vi "LabVIEWSensorDisplayandDrillControlRev1.0.0.vi"() -> ()   [LabVIEW 2020]
uses:
  <vilib>/Instr/_visa.llb/VISA Configure Serial Port (Instr).vi
panel:
  in  "Motor Control Duino":refnum<visa-resource-name>
  out "char sent":string
  in  "Char to Send\na: accelerate\nd: decellerate\ns: stop":string
  in  "Send Data":bool
  in  "stop":bool
  in  "Sensor 2 Byte Count":u32
  in  "Sensor 1 Byte Count":u32
  out "read buffer 2":string
  out "read buffer":string
  in  "Sensor Stop":bool
  out "Current":dbl(knob) scale=0.0..15000.0
  out "RPM":dbl(knob) scale=0.0..15000.0
  in  "Sensor Duino":refnum<visa-resource-name>
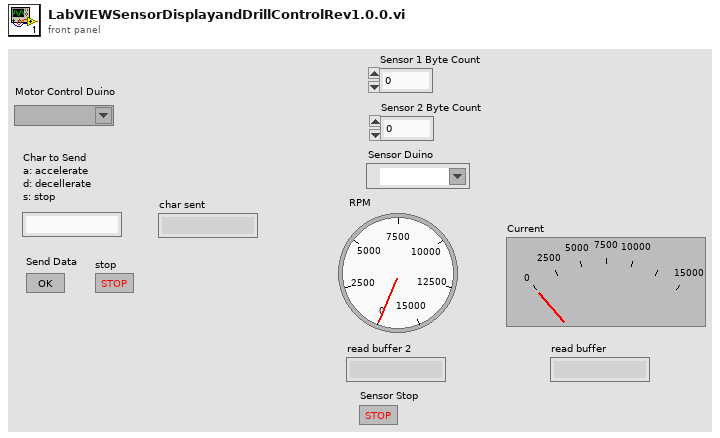
[diagram p1: front panel]
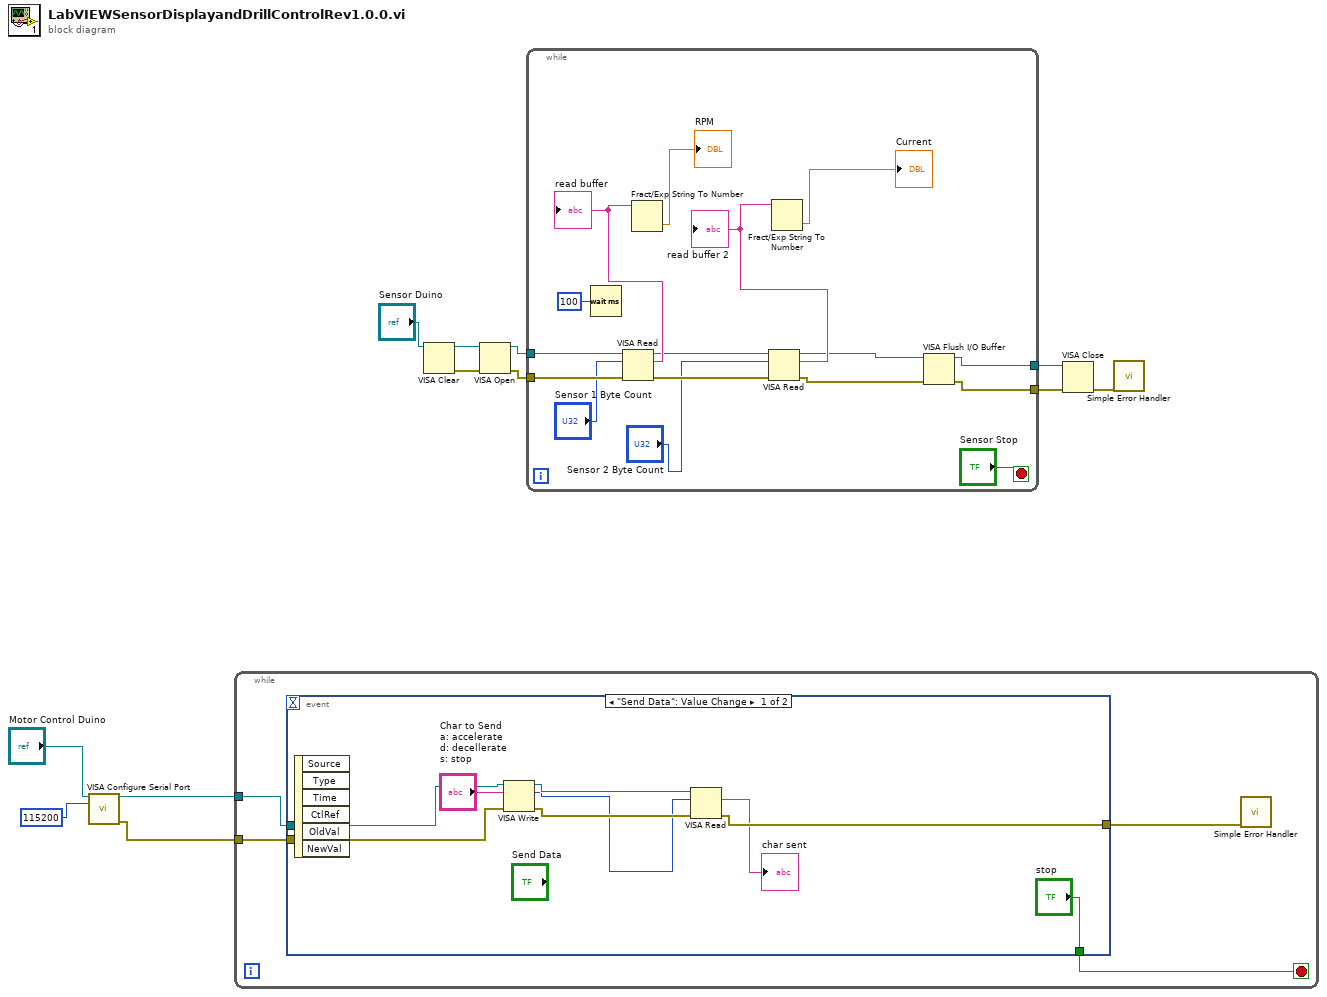
[diagram p0: block diagram]
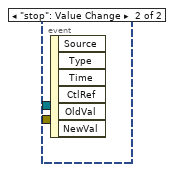
[diagram p2: hidden frame]
diagram:
  n1 = call-poly "VISA Configure Serial Port"("VISA resource name"="Motor Control Duino", "baud rate (9600)"=u32 115200) -> ("VISA resource name out"=w4:refnum<visa-resource-name>, "error out"=w3:errorcluster)  [unwired: 12 in]
  n2 = while {
    tunnel: w4 -> [w15]
    tunnel: w3 -> [w14]
    stop <- w13 stop-if-true
    n3 = event shown="[0] \"Send Data\": Value Change" {
      selector: _ -> [_ _]
      dyn-events: _ -> [_ _]
      timeout: _ -> [_ _]
      tunnel: [w25 _] -> w16
      tunnel: w15 -> [w21 _]
      tunnel: w14 -> [w20 _]
      tunnel: ["stop" _] -> w13
      event "Send Data": Value Change {
        n4 = event-data() -> ()  [unwired: 1 in, 6 out]
        n5 = VISA Write(VISA resource name=w21, write buffer="Char to Send\na: accelerate\nd: decellerate\ns: stop", error in (no error)=w20) -> (VISA resource name out=w23:refnum<visa-resource-name>, return count=w17:u32, error out=w22:errorcluster)
        n6 = VISA Read(VISA resource name=w23, byte count=w17, error in (no error)=w22) -> (read buffer=→"char sent":string, error out=w25:errorcluster)  [unwired: 2 out]
      }
      event "stop": Value Change {
        n7 = event-data() -> ()  [unwired: 1 in, 6 out]
      }
    }
    n8 = call <vilib>:"Simple Error Handler.vi"("error in (no error)"=w16) -> ()  [unwired: 4 in, 5 out]
  }
  n9 = VISA Clear(VISA resource name="Sensor Duino") -> (VISA resource name out=w11:refnum<visa-resource-name>, error out=w12:errorcluster)  [unwired: 1 in]
  n10 = VISA Open(error in (no error)=w12, VISA resource name=w11) -> (VISA resource name=w6:refnum<visa-resource-name>, error out=w5:errorcluster)  [unwired: 3 in]
  n11 = while {
    tunnel: [w32] -> w8
    tunnel: [w31] -> w7
    tunnel: w6 -> [w30]
    tunnel: w5 -> [w29]
    stop <- "Sensor Stop" stop-if-true
    n12 = Wait (ms)(milliseconds to wait=u32 100) -> ()  [unwired: 1 out]
    n13 = VISA Read(VISA resource name=w30, byte count="Sensor 1 Byte Count", error in (no error)=w29) -> (VISA resource name out=w36:refnum<visa-resource-name>, read buffer=w40:string, error out=w35:errorcluster)  [unwired: 1 out]
    "read buffer" <- w40
    n14 = Fract/Exp String To Number(string=w40) -> (number=→"RPM":dbl)  [unwired: 3 in, 1 out]
    n15 = VISA Read(VISA resource name=w36, byte count="Sensor 2 Byte Count", error in (no error)=w35) -> (VISA resource name out=w33:refnum<visa-resource-name>, read buffer=w39:string, error out=w34:errorcluster)  [unwired: 1 out]
    "read buffer 2" <- w39
    n16 = Fract/Exp String To Number(string=w39) -> (number=→"Current":dbl)  [unwired: 3 in, 1 out]
    n17 = VISA Flush I/O Buffer(VISA resource name=w33, error in (no error)=w34) -> (VISA resource name out=w32:refnum<visa-resource-name>, error out=w31:errorcluster)  [unwired: 1 in]
  }
  n18 = VISA Close(VISA resource name=w8, error in (no error)=w7) -> (error out=w9:errorcluster)
  n19 = call <vilib>:"Simple Error Handler.vi"("error in (no error)"=w9) -> ()  [unwired: 4 in, 5 out]
